vi "edtFTPnet_TransferCompletedEx Event Callback.vi"(4 "用户参数":refnum<user-event>, 5 "事件数据":cluster{"sender":refnum<k24>, "e":refnum<k24>}, 6 "控件引用":refnum<k24>, 7 "事件通用数据":cluster{"事件源":i32, "事件类型":u32, "时间标识":u32}) -> ()   [LabVIEW 2013, in "edtFTPnet.lvlib"]
uses:
  edtFTPnet.lvlib
  edtFTPnet.dll
  Ctrls/edtFTPnet_CallbackEvent.ctl
  Ctrls/edtFTPnet_Action.ctl
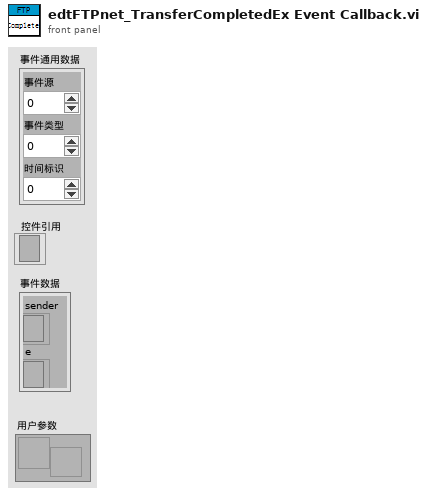
[diagram p1: front panel]
types:
  T1 = typedef "edtFTPnet.lvlib/edtFTPnet_Action.ctl" = enum16{"<None>", "TransferStarted", "Transfering", "TransferCompleted"}
  T2 = typedef "edtFTPnet.lvlib/edtFTPnet_CallbackEvent.ctl" = cluster{"Action":T1, "Direction":i32, "LocalFilePath":string, "RemoteFilename":string}
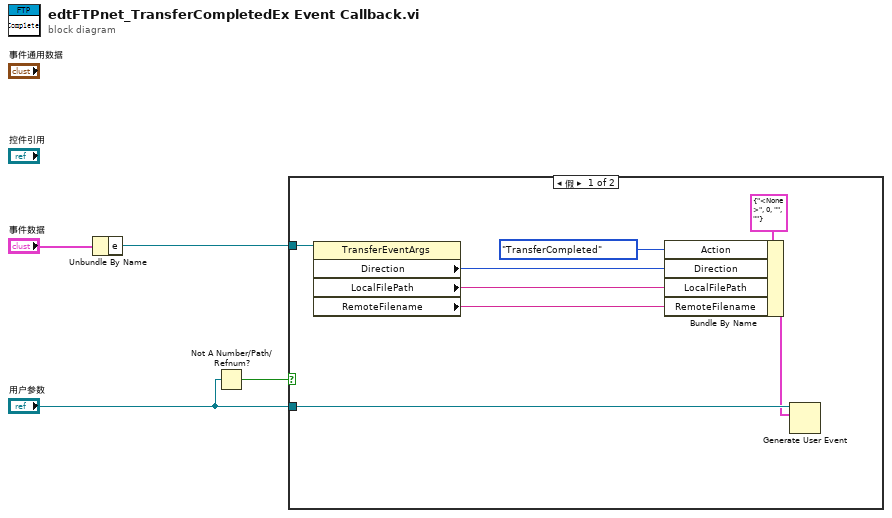
[diagram p0: block diagram]
diagram:
  n1 = Unbundle By Name("事件数据") -> ("e"=w3:refnum<k24>)
  n2 = Not A Number/Path/Refnum?(number/path/refnum="用户参数") -> (NaN/Path/Refnum?=w1:bool)
  n3 = case shown="假" w1 {
    tunnel: w3 -> [w12 _]
    tunnel: "用户参数" -> [w11 _]
    frame False {
      n4 = property class="TransferEventArgs"(reference=w12) -> ("Direction"=w7:i32, "LocalFilePath"=w6:string, "RemoteFilename"=w5:string)  [unwired: 1 in, 2 out]
      n5 = Bundle By Name(cluster=T2 {"Action"=enum."<None>", "Direction"=0, "LocalFilePath"="", "RemoteFilename"=""} ("事件数据"), "Action"=edtFTPnet_Action."TransferCompleted", "Direction"=w7, "LocalFilePath"=w6, "RemoteFilename"=w5) -> (w9:T2)
      n6 = Generate User Event(user event=w11, event data cluster=w9) -> ()  [unwired: 2 in, 2 out]
    }
    frame True {
    }
  }
